vi "Launch Generic Process VI -KTMOD.vi"(6 "Create New Instance if Reentrant (TRUE)":bool=TRUE, 8 "error out":errorcluster, 9 "Process VI FP Control Values to Set":variant[](array[variant]), 10 "Process VI RefNum":variant) -> (0 "error":errorcluster, 1 "Created New Reentrant Instance?":bool, 2 "New Reentrant Instance":refnum<vi>)   [LabVIEW 2020]
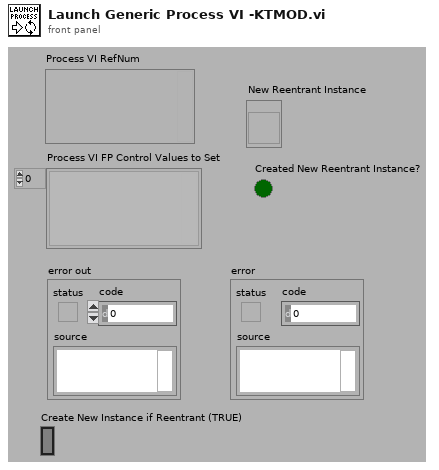
[diagram p1: front panel]
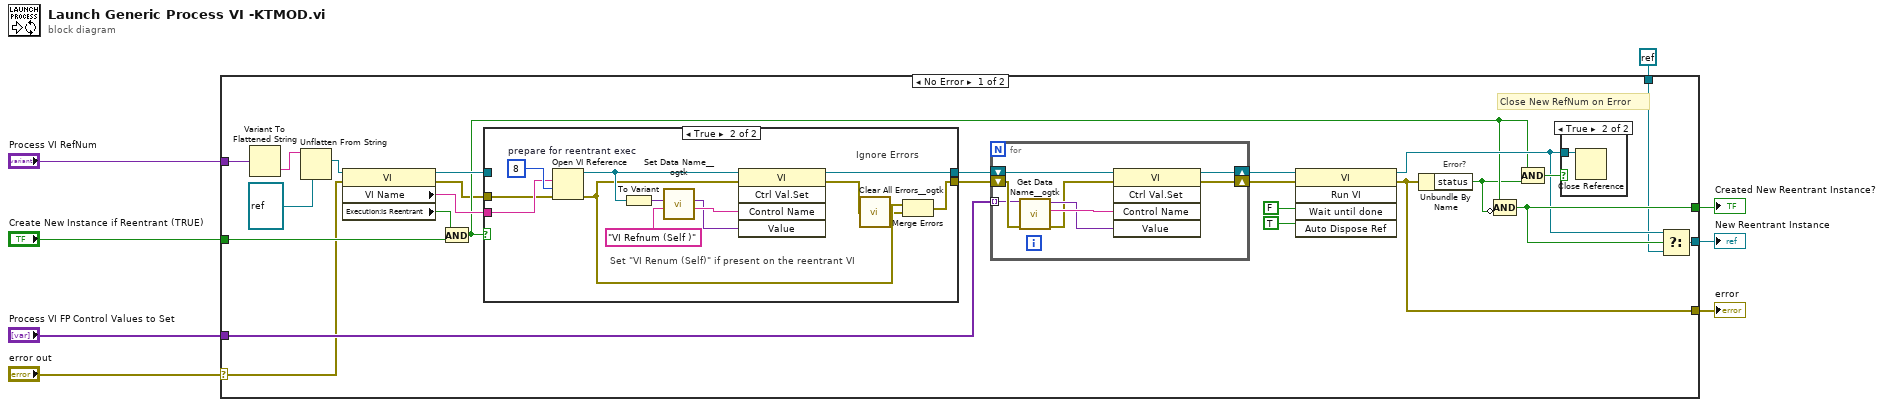
[diagram p0: block diagram]
diagram:
  n1 = case shown="No Error" "error out" {
    selector: "error out" -> [w12 w58]
    tunnel: [w10 w58] -> w8
    tunnel: "Process VI RefNum" -> [w29 _]
    tunnel: "Process VI FP Control Values to Set" -> [w27 _]
    tunnel: [w20 _] -> w4
    tunnel: [w18 w57] -> w3
    tunnel: refnum<k0> refnum -> [w17 w57]
    tunnel: "Create New Instance if Reentrant (TRUE)" -> [w16 _]
    frame No Error {
      # "Error?"
      # "Close New RefNum on Error"
      n2 = Variant To Flattened String(Variant=w29) -> (data string=w26:string)  [unwired: 1 out]
      n3 = Unflatten From String(type=refnum<vi> refnum ("vi reference"), binary string=w26) -> (value=w25:refnum<vi>)  [unwired: 3 in, 2 out]
      n4 = property class="VI"(reference=w25, error in=w12) -> (reference out=w23:refnum<vi>, error out=w11:errorcluster, "VI Name"=w24:string, "Execution:Is Reentrant"=w15:bool)
      n5 = And(x=w15, y=w16) -> (x .and. y?=w14:bool)
      n6 = case shown="True" w14 {
        tunnel: [w36 w42] -> w13
        tunnel: [w35 w38] -> w32
        tunnel: w24 -> [_ w47]
        tunnel: w23 -> [w36 _]
        tunnel: w11 -> [w35 w40]
        frame False {
        }
        frame True {
          w46 = "VI Refnum (Self )" ("Control Name")
          w48 = 8  # prepare for reentrant exec
          # "Set \"VI Renum (Self)\" if present on the reentrant VI"
          # "Ignore Errors"
          n7 = Open VI Reference(vi path=w47, options=w48, error in (no error)=w40) -> (vi reference=w43:refnum<vi>, error out=w39:errorcluster)  [unwired: 3 in]
          n8 = To Variant(anything=w43) -> (Variant=w44:variant)
          n9 = call <userlib>:"Set Data Name__ogtk.vi"("Data Name"=w46, "Data"=w44) -> ("Renamed Data"=w45:variant)  [unwired: 8 in, 1 out]
          n10 = invoke class="VI" method="Ctrl Val.Set"(reference=w43, error in=w39, "Control Name"=w46, "Value"=w45) -> (reference out=w42:refnum<vi>, error out=w41:errorcluster)  [unwired: 1 in, 3 out]
          n11 = call <userlib>:"Clear All Errors__ogtk.vi"("Error In"=w41) -> ("Error Out"=w37:errorcluster)  [unwired: 3 in]
          n12 = Merge Errors(w39, w37) -> (w38:errorcluster)
        }
      }
      n13 = for {
        shift-right: [w54] -> w30
        shift-left: w13 -> [w56]
        shift-right: [w55] -> w31
        shift-left: w32 -> [w50]
        tunnel: w27 -> [w49] mode=indexing
        n14 = call <userlib>:"Get Data Name__ogtk.vi"("error in (no error)"=w50, "Data"=w49) -> ("error out"=w51:errorcluster, "Data Name"=w53:string, "Data dup"=w52:variant)  [unwired: 7 in]
        n15 = invoke class="VI" method="Ctrl Val.Set"(reference=w56, error in=w51, "Control Name"=w53, "Value"=w52) -> (reference out=w54:refnum<vi>, error out=w55:errorcluster)  [unwired: 1 in, 3 out]
      }
      n16 = invoke class="VI" method="Run VI"(reference=w30, error in=w31, "Wait until done"=FALSE, "Auto Dispose Ref"=TRUE) -> (reference out=w19:refnum<vi>, error out=w10:errorcluster)  [unwired: 1 in, 3 out]
      n17 = Unbundle By Name(w10) -> ("status"=w9:bool)
      n18 = Compound Arithmetic op=AND(w14, invert w9) -> (w20:bool)
      n19 = Compound Arithmetic op=AND(w14, w9) -> (w21:bool)
      n20 = case shown="True" w21 {
        tunnel: w19 -> [_ w34]
        frame False {
        }
        frame True {
          n21 = Close Reference(reference=w34) -> ()  [unwired: 1 in, 1 out]
        }
      }
      n22 = Select(t=w19, s=w20, f=w17) -> (s? t:f=w18:refnum<vi>)
    }
    frame Error {
    }
  }
  "error" <- w8
  "New Reentrant Instance" <- w3
  "Created New Reentrant Instance?" <- w4
